vi "Add(I8[]).vi"(1 "Enable(T)":bool=TRUE, 2 "In":i8[](array[numeric]), 4 "n":i8=1) -> (6 "Out":i8[](array[numeric]))   [LabVIEW 2013]
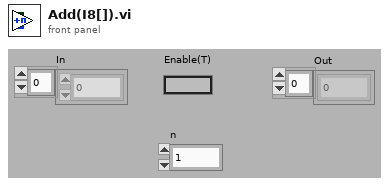
[diagram p1: front panel]
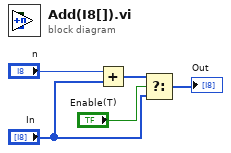
[diagram p0: block diagram]
diagram:
  n1 = Add(x="n", y="In") -> (x+y=w1:i8[])
  n2 = Select(t=w1, s="Enable(T)", f="In") -> (s? t:f=→"Out":i8[])
